vi "0002-01.vi"(11 "sér. (e)":T1) -> (3 "sér. (s)":T1)   [LabVIEW 2010, in "lv_01.lvlib"]
doc: "La série est générée à partir de la commande do_serie."
uses:
  lv_01.lvlib
  do_serie-c.ctl
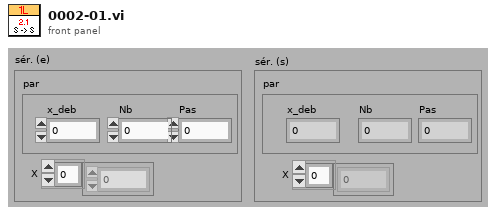
[diagram p1: front panel]
types:
  T1 = typedef "lv_01.lvlib/do_serie-c.ctl" = cluster{"X":dbl[], "par":cluster{"x_deb":dbl, "Pas":dbl, "Nb":dbl}}
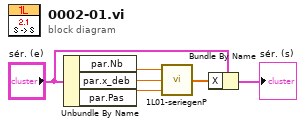
[diagram p0: block diagram]
diagram:
  n1 = Unbundle By Name("sér. (e)") -> ("par.Nb"=w6:dbl, "par.x_deb"=w5:dbl, "par.Pas"=w4:dbl)
  n2 = call "1L01-seriegenP.vi"("Pas"=w4, "x_deb"=w5, "Nb"=w6) -> ("X"=w1:dbl[])
  n3 = Bundle By Name(cluster="sér. (e)", "X"=w1) -> (→"sér. (s)":T1)
